vi "E01.vi"() -> ()   [LabVIEW 2020]
panel:
  in  "Velocidad (ms)":dbl(knob) scale=0.0..100.0
  in  "Botón de paro":bool
  out "Waveform Chart":dbl(graph)
  in  "Gráfica":enum16{"Seno", "Coseno", "Tangente"}(ring)
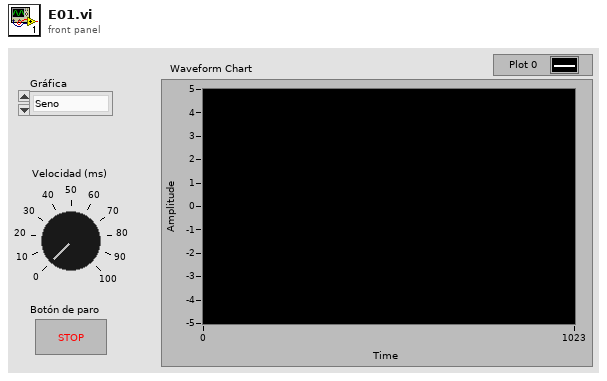
[diagram p1: front panel]
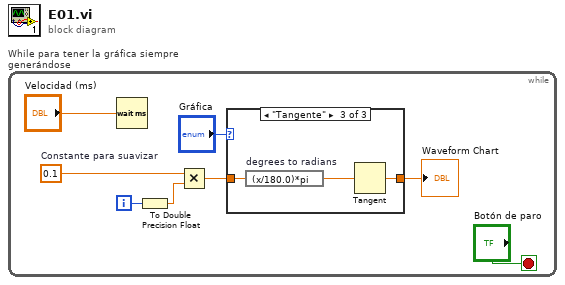
[diagram p0: block diagram]
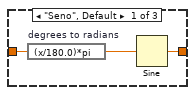
[diagram p2: hidden frame]
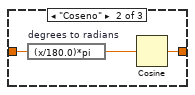
[diagram p3: hidden frame]
diagram:
  n1 = while "While para tener la gráfica siempre generándose" {
    i -> [w2]
    stop <- "Botón de paro" stop-if-true
    w4 = 0.1  # Constante para suavizar
    n2 = Wait (ms)(milliseconds to wait="Velocidad (ms)") -> ()  [unwired: 1 out]
    n3 = To Double Precision Float(number=w2) -> (double precision float=w1:dbl)
    n4 = Multiply(x=w4, y=w1) -> (x*y=w3:dbl)
    n5 = case shown="\"Tangente\"" "Gráfica" {
      tunnel: [w11 w12 w17] -> w6
      tunnel: w3 -> [w10 w14 w16]
      frame "Seno", Default {
        n6 = expression code="(x/180.0)*pi" "degrees to radians"(w10) -> (w9:dbl)
        n7 = Sine(x=w9) -> (sin(x)=w11:dbl)
      }
      frame "Coseno" {
        n8 = expression code="(x/180.0)*pi" "degrees to radians"(w14) -> (w13:dbl)
        n9 = Cosine(x=w13) -> (cos(x)=w12:dbl)
      }
      frame "Tangente" {
        n10 = expression code="(x/180.0)*pi" "degrees to radians"(w16) -> (w15:dbl)
        n11 = Tangent(1:w15) -> (0:w17:dbl)
      }
    }
    "Waveform Chart" <- w6
  }
